vi "get Contact wfm.vi"(0 "reference in":refnum<class "Fcurve.lvclass">, 1 ".Zeroed (wfms.array)":waveform(dbl)[](array[waveform]), 2 "End Index (approach)":i32, 5 "error in (no error)":errorcluster) -> (14 "reference out":refnum<class "Fcurve.lvclass">, 15 "Zeroed (wfms.array) out":waveform(dbl)[](array[waveform]), 16 "Duration":i32, 17 "Contact indices [start,duration]":cluster{"Start":i32, "Duration":i32}, 18 "Contact":cluster{"X":dbl[], "Y":dbl[]}, 19 "error out":errorcluster)   [LabVIEW 2019, in "Fcurve.lvclass"]
uses:
  Fcurve.lvclass
  Fcurve sections.ctl
  <vilib>/Waveform/WDTOps.llb/WDT Get Waveform Subset DBL.vi
panel:
  out "Start":i32
  out "Duration (S)":dbl
  out "Duration":dbl
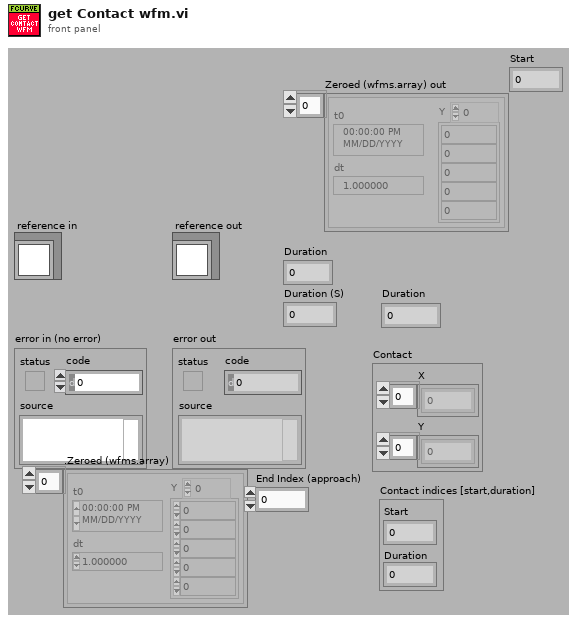
[diagram p1: front panel]
types:
  T1 = typedef "Fcurve.lvclass/Fcurve sections.ctl" = enum16{"Approach", "Contact", "Retract"}
  T2 = typedef "Fcurve.lvclass/ObjectAttributes.ctl" = cluster{"MyAttribute":dbl, "Fcurve Metadata":T3, "Contact Spread of dev":dbl, "Tau Delay (ms)":dbl, "Points of contact":dbl, "Def_wfm":cluster{"Max":dbl, "Min":dbl}, "Zpos_wfm":cluster{"Max":dbl, "Min":dbl}, "Contact stat?":bool, "Real AI dt (s)":dbl, "Decimation":cluster{"App":cluster{"Dec":i32, "apply":bool}, "Con":cluster{"Dec":i32, "apply":bool}, "Ret":cluster{"Dec":i32, "apply":bool}}, "Segment def[0]":dbl, "Segment Zpos[0]":dbl, "Raw Datum":waveform(dbl)[], "Group metadata":T4, "M_data obj":refnum<class "metadata.lvclass">, "Channel name(s)":string[], "Segment fcurve data":cluster{"X":dbl[], "Y":dbl[]}[], "Segment duration":cluster{"Start":i32, "Duration":i32}[], "Segment info":T5[], "Segment durations (S)":dbl[], "Segments Maxmin":T7[]}
  T3 = typedef "Fcurve.lvclass/Metadata.ctl" = cluster{"dt (us)":dbl, "Dec Factor":dbl, "Z piezo Sensitivity (nm/V)":dbl, "K (N/m)":dbl, "Sp (V)":dbl, "Contact (ms)":dbl, "Zpos contact":dbl, "Vel_app (nm/s)":dbl, "Vel_ret (nm/s)":dbl, "deltaV (nm)":dbl, "Def_V0 (v)":dbl, "Piezo gain":dbl, "invOLS (nm/V)":dbl}
  T4 = typedef "TDMS_DataHandler.lvclass/Fcurve Meta data.ctl" = cluster{"property names":string[], "property values":variant[]}
  T5 = typedef "Fcurve.lvclass/Fcurve segments --cluster.ctl" = cluster{"type":T6, "nb points":i32, "dec factor":u32, "sampling rate (S/s)":u32}
  T6 = typedef "metadata.lvclass/Segment type--combobox.ctl" = string
  T7 = typedef "Fcurve.lvclass/Segment MaxMin --cluster.ctl" = cluster{"Def":cluster{"max value":dbl, "min value":dbl}, "Zpos":cluster{"max value":dbl, "min value":dbl}}
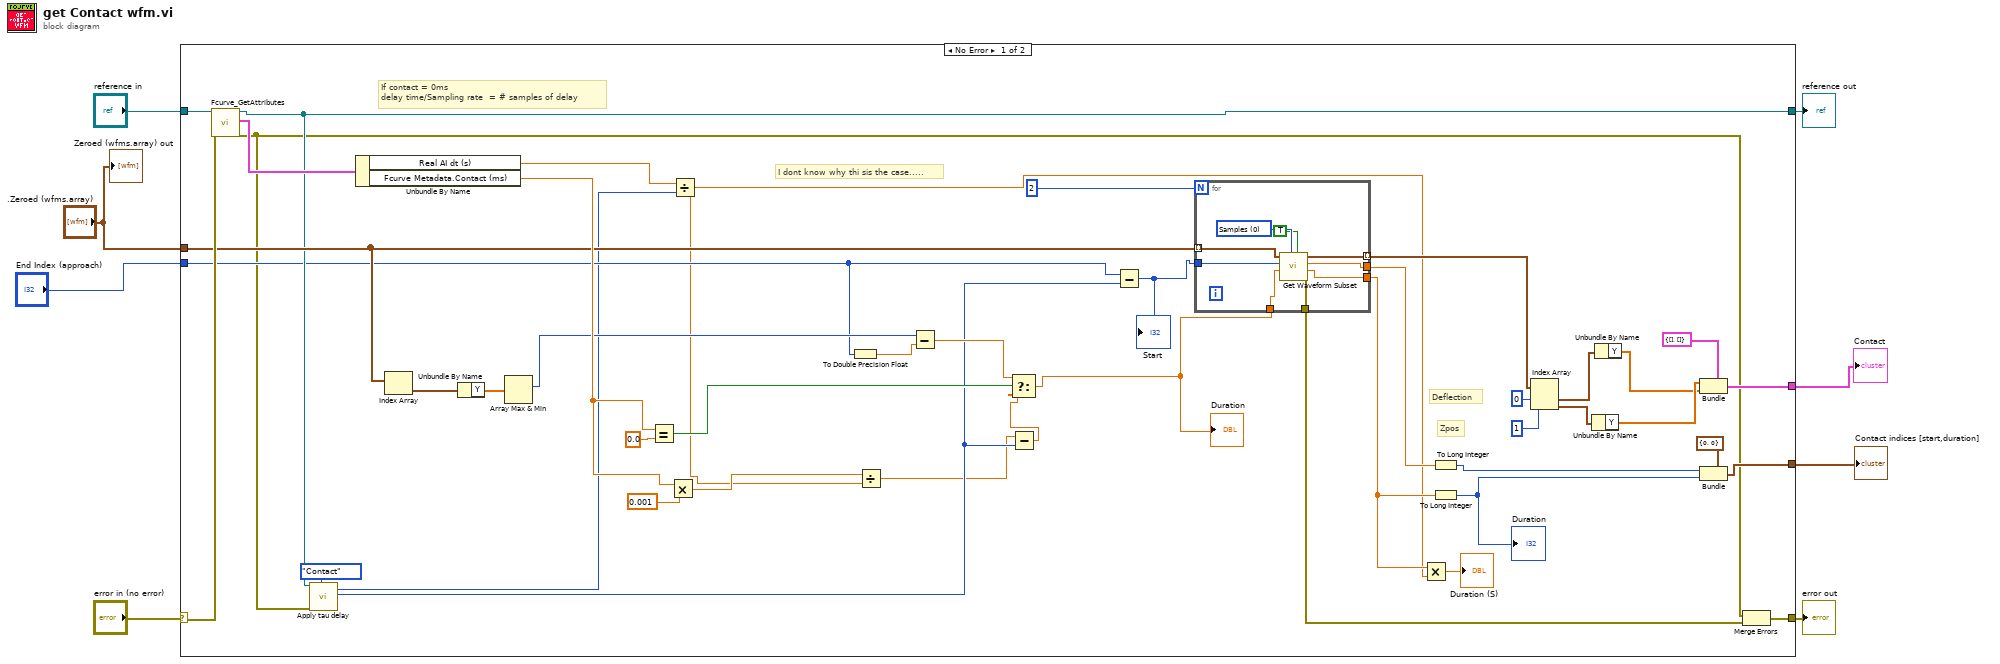
[diagram p0: block diagram]
diagram:
  n1 = case shown="No Error" "error in (no error)" {
    selector: "error in (no error)" -> [w52 w64]
    tunnel: [w53 w64] -> w7
    tunnel: [w22 w63] -> w5
    tunnel: "reference in" -> [w39 w63]
    tunnel: [w35 _] -> w4
    tunnel: [w34 _] -> w3
    tunnel: ".Zeroed (wfms.array)" -> [w28 _]
    tunnel: "End Index (approach)" -> [w21 _]
    frame No Error {
      # "I dont know why thi sis the case....."
      # "Deflection"
      # "Zpos"
      # "If contact = 0ms\ndelay time/Sampling rate  = # samples of delay"
      n2 = call "Fcurve_GetAttributes.vi"("reference in"=w39, "error in (no error)"=w52) -> ("reference out"=w22:refnum<class "Fcurve.lvclass">, "attributes"=w51:T2, "error out"=w15:errorcluster)  [unwired: 14 in, 1 out]
      n3 = call "Apply tau delay.vi"("reference in"=w22, "error in (no error)"=w15, "Section"=Fcurve_sections."Contact") -> ("Dec factor"=w9:i32, "# of samples"=w19:i32)  [unwired: 13 in, 2 out]
      n4 = Unbundle By Name(w51) -> ("Real AI dt (s)"=w16:dbl, "Fcurve Metadata.Contact (ms)"=w32:dbl)
      n5 = Index Array(array=w28) -> (element=w27:waveform(dbl))  [unwired: 1 in]
      n6 = Unbundle By Name(w27) -> ("Y"=w26:dbl[])
      n7 = Array Max & Min(array=w26) -> (max index (indices)=w24:i32)  [unwired: 3 out]
      n8 = Equal?(x=w32, y=0.0) -> (x = y?=w44:bool)
      n9 = Multiply(x=w32, y=0.001) -> (x*y=w31:dbl)
      n10 = Divide(x=w16, y=w9) -> (x/y=w14:dbl)
      n11 = To Double Precision Float(number=w21) -> (double precision float=w25:dbl)
      n12 = Divide(x=w31, y=w14) -> (x/y=w12:dbl)
      n13 = Subtract(x=w24, y=w25) -> (x-y=w23:dbl)
      n14 = Subtract(x=w12, y=w19) -> (x-y=w11:dbl)
      n15 = Select(t=w23, s=w44, f=w11) -> (s? t:f=w13:dbl)
      "Duration" <- w13
      n16 = Subtract(x=w21, y=w19) -> (x-y=w20:i32)
      "Start" <- w20
      n17 = for {
        N: 2 -> [_]
        tunnel: [w61] -> w18
        tunnel: [w60] -> w49 mode=indexing
        tunnel: w28 -> [w59] mode=indexing
        tunnel: w20 -> [w56]
        tunnel: [w57] -> w41
        tunnel: [w55] -> w38
        tunnel: w13 -> [w54]
        w62 = u16 0 items=["Samples", "Relative Time"] ("start/duration format")
        n18 = call-poly <vilib>:"Get Waveform Subset.vi"("open interval? (T)"=TRUE, "start/duration format"=w62, "duration"=w54, "start samples/time"=w56, "waveform in"=w59) -> ("error out"=w55:errorcluster, "actual duration"=w61:dbl, "actual start samples/time"=w57:dbl, "waveform out"=w60:waveform(dbl))  [unwired: 1 in]
      }
      n19 = Multiply(x=w18, y=w14) -> (x*y=→"Duration (S)":dbl)
      n20 = To Long Integer(number=w41) -> (32bit integer=w40:i32)
      n21 = To Long Integer(number=w18) -> (32bit integer=w42:i32)
      "Duration" <- w42
      n22 = Index Array(array=w49, index #1=0 ("index"), index #2=1 ("index")) -> (element #1=w48:waveform(dbl), element #2=w47:waveform(dbl))
      n23 = Unbundle By Name(w47) -> ("Y"=w30:dbl[])
      n24 = Unbundle By Name(w48) -> ("Y"=w29:dbl[])
      n25 = Bundle(cluster=cluster{"X":dbl[], "Y":dbl[]} {"X"=[], "Y"=[]} ("Fcurve.Approach"), "X"=w30, "Y"=w29) -> (w34:cluster{"X":dbl[], "Y":dbl[]})
      n26 = Bundle(cluster=cluster{"Start":i32, "Duration":i32} {"Start"=0, "Duration"=0} ("Fcurve index.Contact indices"), "Start"=w40, "Duration"=w42) -> (w35:cluster{"Start":i32, "Duration":i32})
      n27 = Merge Errors(w15, w38) -> (w53:errorcluster)
    }
    frame Error {
    }
  }
  "error out" <- w7
  "reference out" <- w5
  "Contact indices [start,duration]" <- w4
  "Contact" <- w3
  "Zeroed (wfms.array) out" <- ".Zeroed (wfms.array)"
